vi "myPython.vi"() -> ()   [LabVIEW 2019]
panel:
  in  "Tab Control":T1(tab)
  in  "a":dbl=41.0
  in  "b":dbl=1.0
  out "a + b":dbl
  in  "a 3":dbl=41.0
  in  "b 3":dbl=1.0
  out "a + b 2":dbl
  in  "b":i32=1
  in  "a":i32=41
  out "a + b":i32
  in  "array":i32[](array[numeric])=[1, 2, 3]
  in  "new element":i32=4
  out "modified array":i32[](array[numeric])
  in  "str1":string="Hello "
  in  "str2":string="World"
  out "concatenated string":string
  in  "a 2":dbl[][](array[numeric])=[[1.0, 2.0, 3.0], [4.0, 5.0, 6.0], [7.0, 8.0, 9.0]]
  in  "b 2":dbl[][](array[numeric])=[[1.0, 0.0, 0.0], [0.0, 1.0, 0.0], [0.0, 0.0, 1.0]]
  out "a*b":dbl[][](array[numeric])
  out "<JSON>":string
  out "result":i32[](array[numeric])
  in  "Numeric":i32=100 format="%.0p"
  out "create JSON":dbl format="%#_6p"
  out "parse JSON":dbl format="%#_6p"
  out "open Python session":dbl format="%#_6p"
  out "error out":errorcluster
  in  "error in (no error)":errorcluster
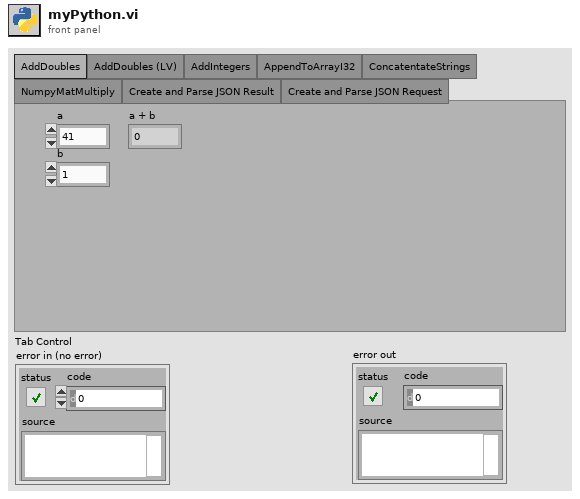
[diagram p1: front panel]
types:
  T1 = enum32{"AddDoubles", "AddDoubles (LV)", "AddIntegers", "AppendToArrayI32", "ConcatentateStrings", "NumpyMatMultiply", "Create and Parse JSON Result", "Create and Parse JSON Request"}
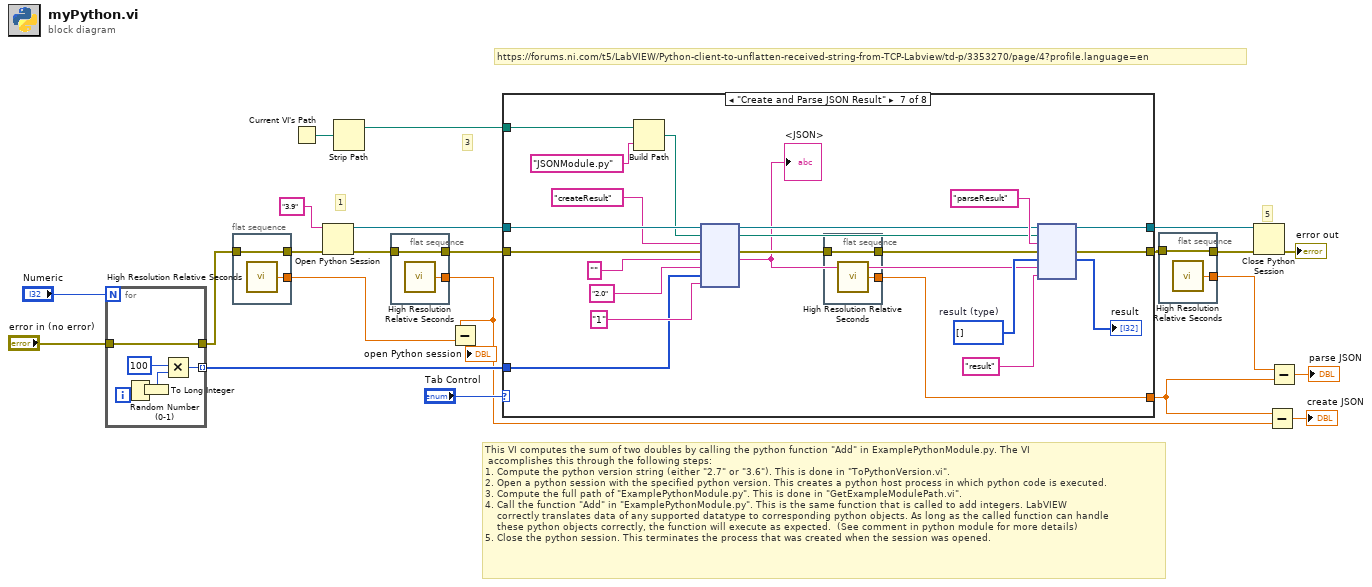
[diagram p0: block diagram]
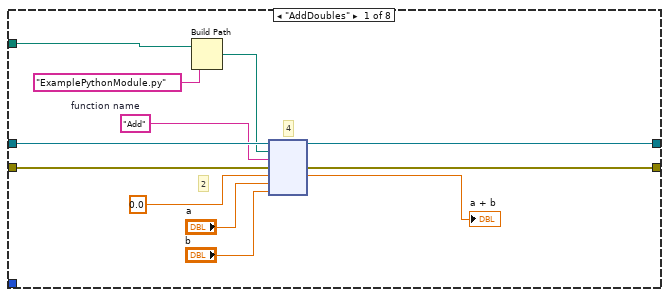
[diagram p2: hidden frame]
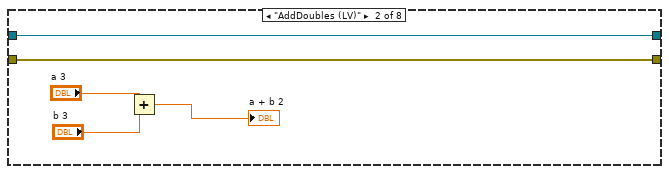
[diagram p3: hidden frame]
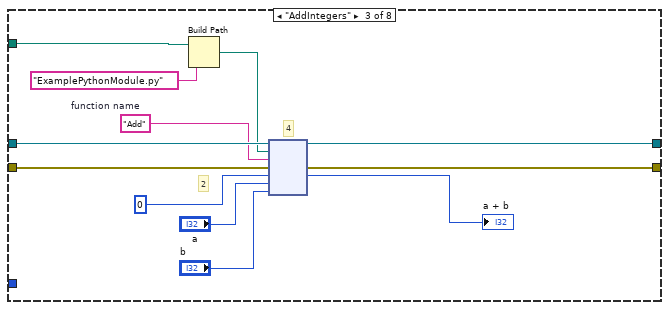
[diagram p4: hidden frame]
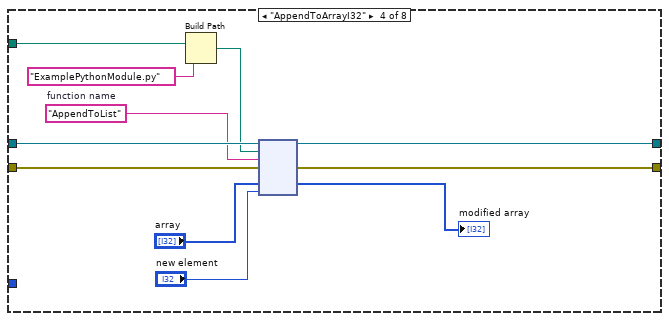
[diagram p5: hidden frame]
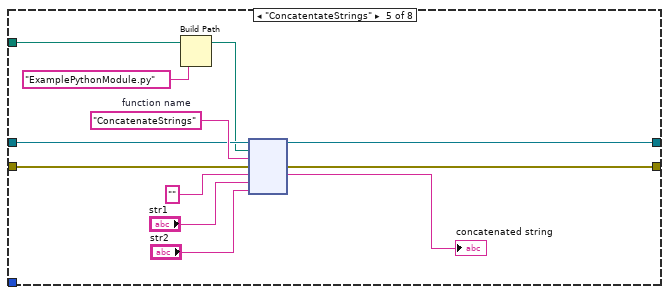
[diagram p6: hidden frame]
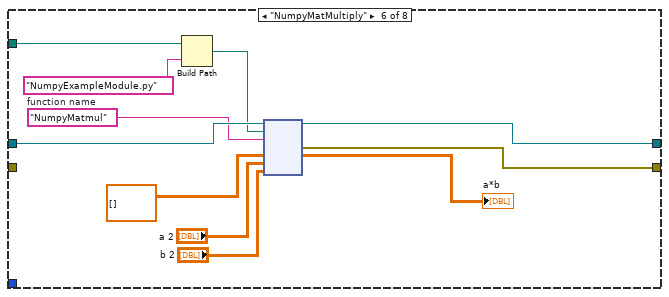
[diagram p7: hidden frame]
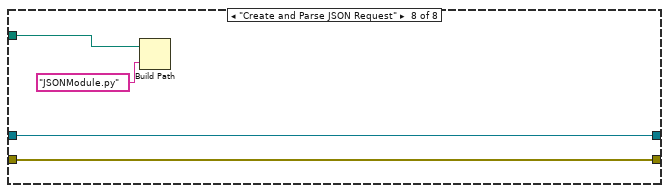
[diagram p8: hidden frame]
diagram:
  # "https://forums.ni.com/t5/LabVIEW/Python-client-to-unflatten-received-string-from-TCP-Labview/td-p/3353270/page/4?profile.language=en"
  # "5"
  # "3"
  # "1"
  # "This VI computes the sum of two doubles by calling the python function \"Add\" in ExamplePythonModule.py. The VI\n accomplishes this through the following steps:\n1. Compute the python version string (either \"2.7\" or \"3.6\"). This is done in \"ToPythonVersion.vi\". \n2. Open a python session with the specified python version. This creates a python host process in which python code is executed.\n3. Compute the full path of \"ExamplePythonModule.py\". This is done in \"GetExampleModulePath.vi\".\n4. Call the function \"Add\" in \"ExamplePythonModule.py\". This is the same function that is called to add integers. LabVIEW \n    correctly translates data of any supported datatype to corresponding python objects. As long as the called function can handle\n    these python objects correctly, the function will execute as expected.  (See comment in python module for more details)\n5. Close the python session. This terminates the process that was created when the session was opened."
  n1 = for {
    N: "Numeric" -> [_]
    tunnel: [w27] -> w12 mode=indexing
    tunnel: "error in (no error)" -> [w25]
    tunnel: [w25] -> w3
    n2 = Random Number (0-1)() -> (number: 0 to 1=w26:dbl)
    n3 = To Long Integer(number=w26) -> (32bit integer=w24:i32)
    n4 = Multiply(x=100, y=w24) -> (x*y=w27:i32)
  }
  n5 = flat-sequence {
    tunnel: [w30] -> w6
    tunnel: w3 -> [w30]
    tunnel: [w29] -> w4
    frame #0 {
      n6 = call <vilib>:"High Resolution Relative Seconds.vi"() -> ("relative seconds"=w29:dbl)
    }
  }
  n7 = Current VI's Path() -> (path=w22:path)
  n8 = Open Python Session(python version="3.9" ("Python version"), 3:w6) -> (session out=w15:refnum<k35>, error out=w18:errorcluster)  [unwired: 1 in]
  n9 = Strip Path(path=w22) -> (stripped path=w20:path)  [unwired: 1 out]
  n10 = flat-sequence {
    tunnel: [w32] -> w19
    tunnel: w18 -> [w32]
    tunnel: [w31] -> w7
    frame #0 {
      n11 = call <vilib>:"High Resolution Relative Seconds.vi"() -> ("relative seconds"=w31:dbl)
    }
  }
  n12 = Subtract(x=w7, y=w4) -> (x-y=→"open Python session":dbl)
  n13 = case shown="\"Create and Parse JSON Result\"" "Tab Control" {
    tunnel: w15 -> [w44 w48 w61 w72 w80 w93 w113 w118]
    tunnel: w19 -> [w43 w49 w60 w71 w79 _ w112 w119]
    tunnel: [w41 w48 w58 w65 w77 w92 w104 w118] -> w13
    tunnel: [w40 w49 w57 w66 w78 w91 w105 w119] -> w14
    tunnel: w20 -> [w34 _ w51 w63 w75 w85 w114 w120]
    tunnel: w12 -> [_ _ _ _ _ _ w103 _]
    tunnel: [_ _ _ _ _ _ w96 _] -> w8
    frame "AddDoubles" {
      w42 = "Add"  # function name
      # "4"
      # "2"
      n14 = Build Path(base path=w34, name or relative path="ExamplePythonModule.py") -> (appended path=w33:path)
      n15 = node(w44, w33, w42, w43, 0.0 ("a"), "a", "b") -> (w41:refnum<k35>, w40:errorcluster, →"a + b":dbl)  [unwired: 2 in, 2 out]
    }
    frame "AddDoubles (LV)" {
      n16 = Add(x="a 3", y="b 3") -> (x+y=→"a + b 2":dbl)
    }
    frame "AddIntegers" {
      w59 = "Add"  # function name
      # "4"
      # "2"
      n17 = Build Path(base path=w51, name or relative path="ExamplePythonModule.py") -> (appended path=w50:path)
      n18 = node(w61, w50, w59, w60, 0 ("a"), "a", "b") -> (w58:refnum<k35>, w57:errorcluster, →"a + b":i32)  [unwired: 2 in, 2 out]
    }
    frame "AppendToArrayI32" {
      w70 = "AppendToList"  # function name
      n19 = Build Path(base path=w63, name or relative path="ExamplePythonModule.py") -> (appended path=w62:path)
      n20 = node(w72, w62, w70, w71, "array", "new element") -> (w65:refnum<k35>, w66:errorcluster, →"modified array":i32[])  [unwired: 3 in, 2 out]
    }
    frame "ConcatentateStrings" {
      w83 = "ConcatenateStrings"  # function name
      n21 = Build Path(name or relative path="ExamplePythonModule.py") -> ()  [unwired: 1 in, 1 out]
      n22 = node(w80, w75, w83, w79, "" ("str1"), "str1", "str2") -> (w77:refnum<k35>, w78:errorcluster, →"concatenated string":string)  [unwired: 2 in, 2 out]
    }
    frame "NumpyMatMultiply" {
      w87 = "NumpyMatmul"  # function name
      n23 = Build Path(base path=w85, name or relative path="NumpyExampleModule.py") -> (appended path=w84:path)
      n24 = node(w93, w84, w87, dbl[][] [] ("b"), "a 2", "b 2") -> (w92:refnum<k35>, w91:errorcluster, →"a*b":dbl[][])  [unwired: 3 in, 2 out]
    }
    frame "Create and Parse JSON Result" {
      w101 = i32[] []  # result (type)
      n25 = Build Path(base path=w114, name or relative path="JSONModule.py") -> (appended path=w106:path)
      n26 = node(w113, w106, "createResult" ("name or relative path"), w112, "", "2.0", w103, "1") -> (w107:refnum<k35>, w98:errorcluster, w95:string)  [unwired: 3 in, 2 out]
      "<JSON>" <- w95
      n27 = flat-sequence {
        tunnel: [w117] -> w97
        tunnel: w98 -> [w117]
        tunnel: [w116] -> w96
        frame #0 {
          n28 = call <vilib>:"High Resolution Relative Seconds.vi"() -> ("relative seconds"=w116:dbl)
        }
      }
      n29 = node(w107, w106, "parseResult" ("name or relative path"), w97, w101, w95, "result") -> (w104:refnum<k35>, w105:errorcluster, →"result":i32[])  [unwired: 2 in, 2 out]
    }
    frame "Create and Parse JSON Request" {
      n30 = Build Path(base path=w120, name or relative path="JSONModule.py") -> ()  [unwired: 1 out]
    }
  }
  n31 = flat-sequence {
    tunnel: [w123] -> w17
    tunnel: w14 -> [w123]
    tunnel: [w122] -> w9
    frame #0 {
      n32 = call <vilib>:"High Resolution Relative Seconds.vi"() -> ("relative seconds"=w122:dbl)
    }
  }
  n33 = Close Python Session(session in=w13, error in=w17) -> (11:→"error out":errorcluster)
  n34 = Subtract(x=w8, y=w7) -> (x-y=→"create JSON":dbl)
  n35 = Subtract(x=w9, y=w8) -> (x-y=→"parse JSON":dbl)
